vi "Convert Cluster To Description.vi"(8 "Description Cluster":T1, 9 "error in (no error)":errorcluster) -> (0 "Description String (empty)":string, 1 "error out":errorcluster)   [LabVIEW 2014]
doc: "<b>VI Description:</b> This VI collapses the separate elements of a VI documenation block into a single string with appropriate identifying names. \n<b>VI Version:</b> 1.1.38.Reviewed \n<b>Review Date:</b> 03/09/2012 \n<b>Author:</b> Jason Willis, Ryan Podsim \n<b>Copyright:</b> Copyright © 2010-2014"
uses:
  TYPE_Description Cluster.ctl
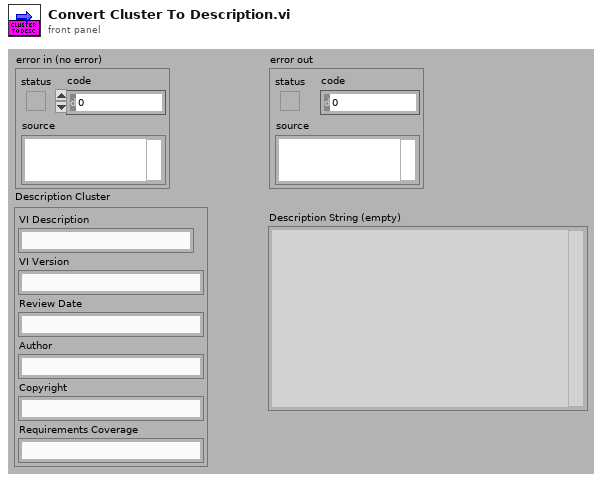
[diagram p1: front panel]
types:
  T1 = typedef "TYPE_Description Cluster.ctl" = cluster{"VI Description":string, "VI Version":string, "Review Date":string, "Author":string, "Copyright":string, "Requirements Coverage":string}
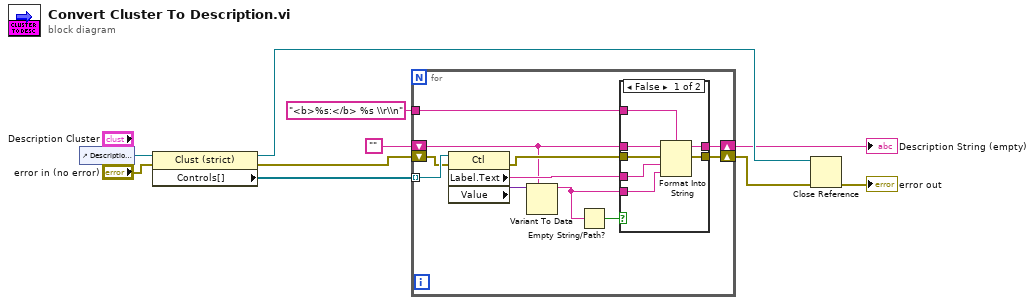
[diagram p0: block diagram]
diagram:
  n1 = control-ref of="Description Cluster"() -> (w6:refnum<vi>)
  n2 = property class="Clust (strict)"(reference=w6, error in="error in (no error)") -> (reference out=w7:refnum<vi>, error out=w9:errorcluster, "Controls[]"=w10:refnum<vi>[])
  n3 = for {
    tunnel: w10 -> [w21] mode=indexing
    shift-right: [w19] -> w2
    shift-left: "" -> [w14]
    tunnel: "<b>%s:</b> %s \\r\\n" ("format string") -> [w13]
    shift-right: [w17] -> w8
    shift-left: w9 -> [w20]
    n4 = property class="Ctl"(reference=w21, error in=w20) -> (error out=w18:errorcluster, "Label.Text"=w16:string, "Value"=w15:variant)  [unwired: 1 out]
    n5 = Variant To Data(type=w14, Variant=w15) -> (data=w11:string)  [unwired: 1 in, 1 out]
    n6 = Empty String/Path?(string/path=w11) -> (empty?=w12:bool)
    n7 = case shown="False" w12 {
      tunnel: [w28 w30] -> w19
      tunnel: w18 -> [w27 w29]
      tunnel: [w26 w29] -> w17
      tunnel: w16 -> [w25 _]
      tunnel: w11 -> [w24 _]
      tunnel: w14 -> [w23 w30]
      tunnel: w13 -> [w22 _]
      frame False {
        n8 = Format Into String(format string=w22, initial string=w23, error in=w27, w25, w24) -> (resulting string=w28:string, error out=w26:errorcluster)
      }
      frame True {
      }
    }
  }
  "Description String (empty)" <- w2
  n9 = Close Reference(reference=w7, error in (no error)=w8) -> (error out=→"error out":errorcluster)
